vi "Trail_Data_Save.vi"(5 "Status":string, 6 "error in (no error)":errorcluster, 7 "RFID":string, 8 "Query":string, 9 "Ref in":T1={"MS SQL Connection"=refnum, "UDL File"=path "", "Time"="", "DCODE"="", "WIP+1"=0, "MC No?"=0, "POKAYOKE?"=FALSE, "Expected Result"="", "Result [Status]"="", "Clock"=0.0, "RFID"="", "WIP Queue"=refnum, "TS Parameter"={"ProfitCenterCode"="", "LineCode"="", "WorkOrderNumber"="", "Model"="", "Model_with_Prefix"="", "VendorCode"="", "SetParameterDateCode"="", "PokaYoke"=0, "Target"=1, "Live_DateCode"="", "CustomerPartNumber"="", "Hand"="", "sBarcode"=FALSE, "FCA"=0, "Ent_Stamp"=timestamp(0 s since 1904-01-01), "STS_CD"=0.0}, "Data_Queue"=[], "RFID Serial No."=""} {"TS Parameter"."FCA" format="%01d"; "TS Parameter"."Target" min=1 max=100000; "TS Parameter"."PokaYoke" min=0 max=1}) -> (0 "error out":errorcluster, 1 "Message":picture, 2 "Saved?":bool, 3 "Ref Out":T1={"MS SQL Connection"=refnum, "UDL File"=path "", "Time"="", "DCODE"="", "WIP+1"=0, "MC No?"=0, "POKAYOKE?"=FALSE, "Expected Result"="", "Result [Status]"="", "Clock"=0.0, "RFID"="", "WIP Queue"=refnum, "TS Parameter"={"ProfitCenterCode"="", "LineCode"="", "WorkOrderNumber"="", "Model"="", "Model_with_Prefix"="", "VendorCode"="", "SetParameterDateCode"="", "PokaYoke"=0, "Target"=1, "Live_DateCode"="", "CustomerPartNumber"="", "Hand"="", "sBarcode"=FALSE, "FCA"=0, "Ent_Stamp"=timestamp(0 s since 1904-01-01), "STS_CD"=0.0}, "Data_Queue"=[], "RFID Serial No."=""} {"TS Parameter"."FCA" format="%01d"; "TS Parameter"."Target" min=1 max=100000; "TS Parameter"."PokaYoke" min=0 max=1})   [LabVIEW 2020]
uses:
  Controls/TD SQL.ctl
  <vilib>/addons/database/Connection.llb/Conn ObjectReference.ctl
  Controls/WIP_State.ctl
  Controls/TS_Parameter.ctl
  Controls/Msg_Type.ctl
  <vilib>/addons/database/NI_Database_API.lvlib
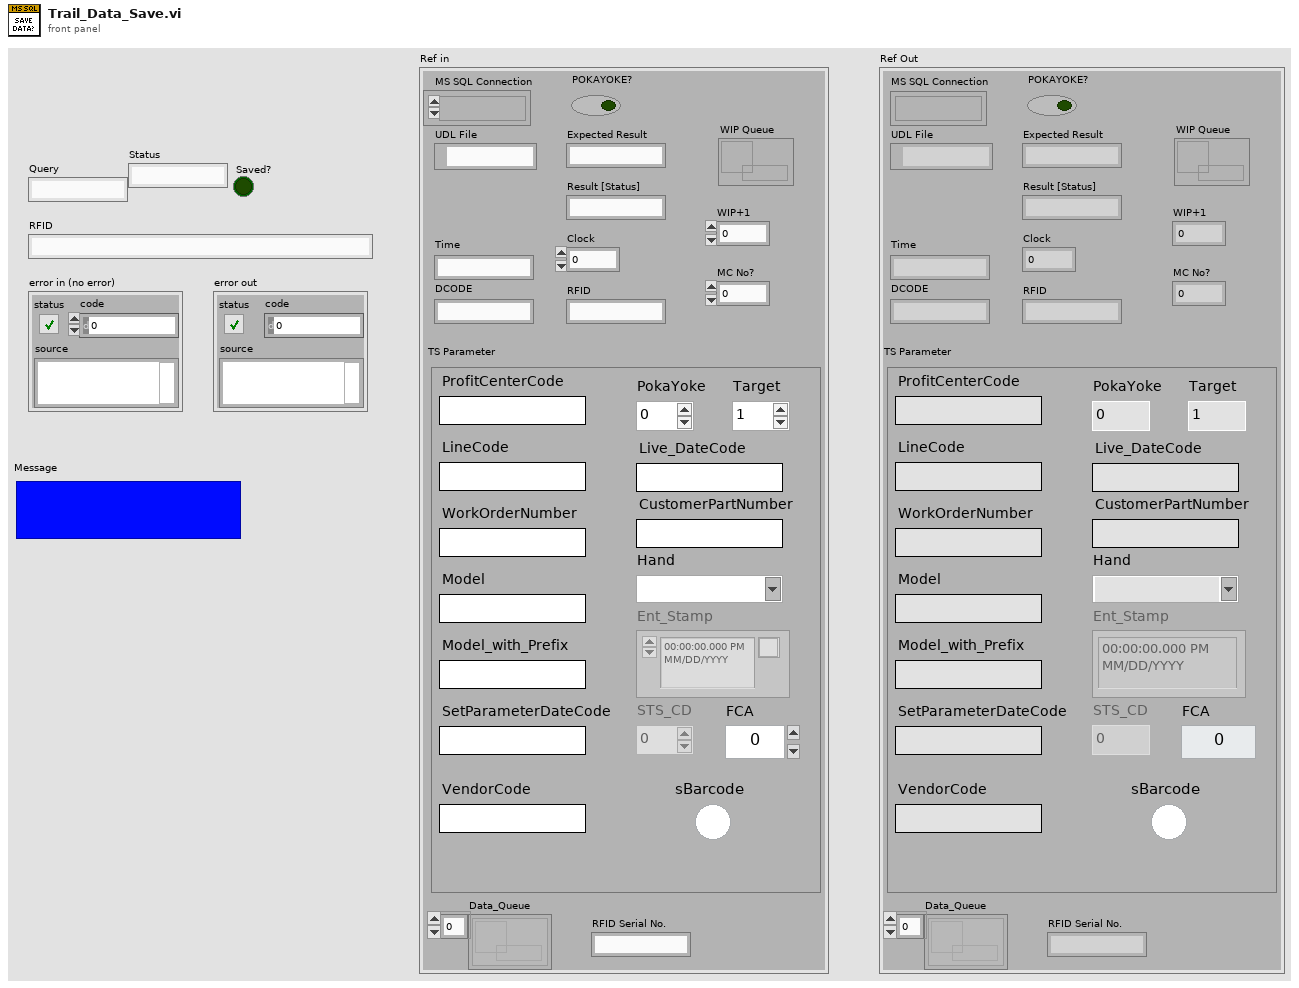
[diagram p1: front panel]
types:
  T1 = typedef "TD SQL.ctl" = cluster{"MS SQL Connection":T2, "UDL File":path, "Time":string, "DCODE":string, "WIP+1":i64, "MC No?":i32, "POKAYOKE?":bool, "Expected Result":string, "Result [Status]":string, "Clock":dbl, "RFID":string, "WIP Queue":refnum<queue>, "TS Parameter":T3, "Data_Queue":refnum<queue>[], "RFID Serial No.":string}
  T2 = typedef "NI_Database_API.lvlib/Conn ObjectReference.ctl" = refnum<k1>
  T3 = typedef "TS_Parameter.ctl" = cluster{"ProfitCenterCode":string, "LineCode":string, "WorkOrderNumber":string, "Model":string, "Model_with_Prefix":string, "VendorCode":string, "SetParameterDateCode":string, "PokaYoke":i32, "Target":i32, "Live_DateCode":string, "CustomerPartNumber":string, "Hand":string, "sBarcode":bool, "FCA":i32, "Ent_Stamp":timestamp, "STS_CD":dbl}
  T4 = typedef "Msg_Type.ctl" = enum16{"Normal", "Pass", "Fail", "Fault", "User", "Bypass", "Fail Save"}
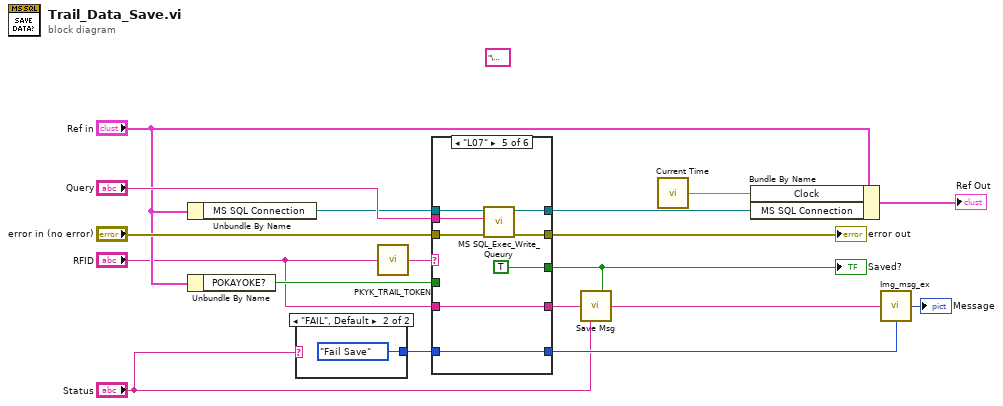
[diagram p0: block diagram]
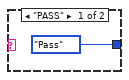
[diagram p2: hidden frame]
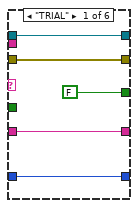
[diagram p3: hidden frame]
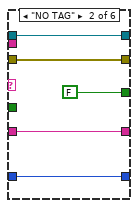
[diagram p4: hidden frame]
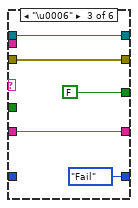
[diagram p5: hidden frame]
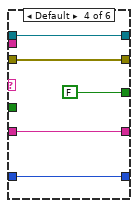
[diagram p6: hidden frame]
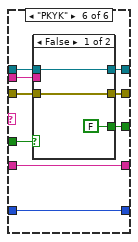
[diagram p7: hidden frame]
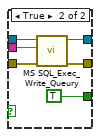
[diagram p8: hidden frame]
diagram:
  (unwired) "\u0006" ("OP20 : Continuity")
  n1 = Unbundle By Name("Ref in") -> ("MS SQL Connection"=w11:T2)
  n2 = Unbundle By Name("Ref in") -> ("POKAYOKE?"=w10:bool)
  n3 = case shown="\"FAIL\", Default" "Status" {
    tunnel: [Msg_Type."Pass" ("Msg Type") Msg_Type."Fail Save" ("Msg Type")] -> w2
    frame "PASS" {
    }
    frame "FAIL", Default {
    }
  }
  n4 = call "PKYK_TRAIL_TOKEN.vi"("RFID In"="RFID") -> ("PKYK?TRAIL"=w15:string)
  n5 = case shown="\"L07\"" w15 {
    tunnel: [w24 w29 w34 w39 w48 w57] -> w16
    tunnel: [w25 w30 w35 w40 w47 w56] -> w9
    tunnel: "error in (no error)" -> [w24 w29 w34 w39 w46 w55]
    tunnel: w11 -> [w25 w30 w35 w40 w45 w54]
    tunnel: "Query" -> [_ _ _ _ w44 w53]
    tunnel: [FALSE FALSE FALSE FALSE TRUE w52] -> w13
    tunnel: w10 -> [_ _ _ _ _ w51]
    tunnel: [w22 w27 w32 w37 w42 w50] -> w5
    tunnel: "RFID" -> [w22 w27 w32 w37 w42 w50]
    tunnel: [w21 w26 Msg_Type."Fail" ("Msg Type") w36 w41 w49] -> w4
    tunnel: w2 -> [w21 w26 _ w36 w41 w49]
    frame "TRIAL" {
    }
    frame "NO TAG" {
    }
    frame "\u0006" {
    }
    frame Default {
    }
    frame "L07" {
      n6 = call "MS SQL_Exec_Write_Queury.vi"("error in (no error)"=w46, "Query"=w44, "Refnum in"=w45) -> ("error out"=w48:errorcluster, "Refnum out"=w47:T2)  [unwired: 7 in]
    }
    frame "PKYK" {
      n7 = case shown="False" w51 {
        tunnel: [w59 w66] -> w57
        tunnel: [w60 w65] -> w56
        tunnel: w55 -> [w59 w64]
        tunnel: w54 -> [w60 w63]
        tunnel: w53 -> [_ w62]
        tunnel: [FALSE TRUE] -> w52
        frame False {
        }
        frame True {
          n8 = call "MS SQL_Exec_Write_Queury.vi"("error in (no error)"=w64, "Query"=w62, "Refnum in"=w63) -> ("error out"=w66:errorcluster, "Refnum out"=w65:T2)  [unwired: 7 in]
        }
      }
    }
  }
  "Saved?" <- w13
  "error out" <- w16
  n9 = call "Save Msg.vi"("Saved?"=w13, "RFID"=w5, "RESULT"="Status") -> ("Message"=w14:string)  [unwired: 12 in]
  n10 = call <userlib>:"Current Time.vi"() -> ("Current Time (Sec)"=w3:dbl)  [unwired: 15 in]
  n11 = Bundle By Name(cluster="Ref in", "Clock"=w3, "MS SQL Connection"=w9) -> (→"Ref Out":T1)
  n12 = call "Img_msg_ex.vi"("Msg Type"=w4, "Message In"=w14) -> ("Message"=→"Message":picture)  [unwired: 2 in]
